vi "NewtonsPSM_Conf_Streaming.vi"(0 "VISA session":refnum<visa-resource-name>, 2 "Interval (1)":dbl=0.9999999999999992 min=0.001 max=10.0 step=0.001, 11 "error in (no error)":errorcluster) -> (4 "dup VISA session":refnum<visa-resource-name>, 15 "error out":errorcluster)   [LabVIEW 2025, in "NewtonsPSM1735.lvlib"]
doc: "This VI set the Datalo mode parameter and selection the paramters to datalog."
uses:
  NewtonsPSM1735.lvlib
panel:
  in  "Parameter (In Phase)":u16(ring) items=["In Phase", "Quadrature", "Tan d", "Magnitude", "Phase", "In-Phase Ratio", "RMS", "RMS2/RMS1", "LVDT Diff", "LVDT Ratio"]
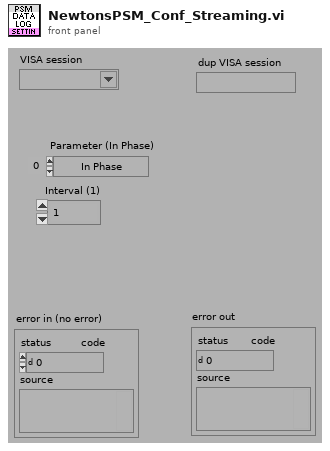
[diagram p1: front panel]
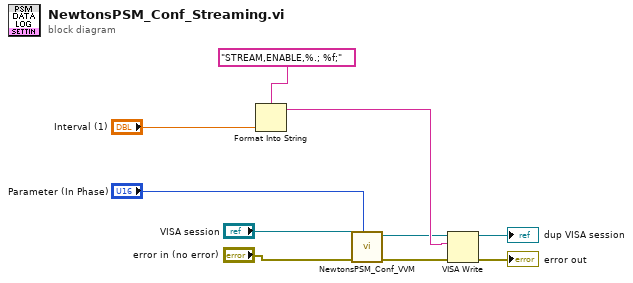
[diagram p0: block diagram]
diagram:
  n1 = Format Into String(format string="STREAM,ENABLE,%.; %f;", "Interval (1)") -> (resulting string=w6:string)  [unwired: 2 in, 1 out]
  n2 = call "NewtonsPSM_Conf_VVM.vi"("Parameter (In Phase)"="Parameter (In Phase)", "error in (no error)"="error in (no error)", "VISA session"="VISA session") -> ("error out"=w3:errorcluster, "dup VISA session"=w1:refnum<visa-resource-name>)  [unwired: 4 in, 3 out]
  n3 = VISA Write(VISA resource name=w1, write buffer=w6, error in (no error)=w3) -> (VISA resource name out=→"dup VISA session":refnum<visa-resource-name>, error out=→"error out":errorcluster)  [unwired: 1 out]
